vi "Slant.vi"(11 "GIC Input":T1={"     Use ?\nOff       On"=[FALSE, TRUE, FALSE, TRUE], "Mode:"=FALSE, "Extra Port"="", "Hokuyo Port"="COM7", "Tx Prop  Port"="COM6", "Compass Port"="", "GPS Port"="", "Num of WPs"=0, "WP Lats and Longs"={"WP Lats"=[], "WP Longs"=[]}, "Obst Lats and Longs"={"Obst Lats"=[], "Obst Longs"=[]}, "Parameters"=[], "GPS Data"=[], "Compass"=0.0, "LMS Vector"=[], "Vision Vector"=[], "Direction Cmd"=0.0, "Speed Cmd"=0.0, "WP Vector"=[], "WP Number"=0, "Extra"=0, "SW Map"=[], "Path Cluster"={"Path x node"=[], "Path y node"=[]}, "Sim Course"=[]} {"Obst Lats and Longs"."Obst Longs" format="%#_8g"; "Obst Lats and Longs"."Obst Lats" format="%#_8g"}) -> (3 "GIC Output":T1={"     Use ?\nOff       On"=[FALSE, TRUE, FALSE, TRUE], "Mode:"=FALSE, "Extra Port"="", "Hokuyo Port"="COM7", "Tx Prop  Port"="COM6", "Compass Port"="", "GPS Port"="", "Num of WPs"=0, "WP Lats and Longs"={"WP Lats"=[], "WP Longs"=[]}, "Obst Lats and Longs"={"Obst Lats"=[], "Obst Longs"=[]}, "Parameters"=[], "GPS Data"=[], "Compass"=0.0, "LMS Vector"=[], "Vision Vector"=[], "Direction Cmd"=0.0, "Speed Cmd"=0.0, "WP Vector"=[], "WP Number"=0, "Extra"=0, "SW Map"=[], "Path Cluster"={"Path x node"=[], "Path y node"=[]}, "Sim Course"=[]} {"Obst Lats and Longs"."Obst Longs" format="%#_8g"; "Obst Lats and Longs"."Obst Lats" format="%#_8g"})   [LabVIEW 2014]
panel:
  out "test1":dbl
  out "yy":dbl
  out "ll":dbl
  out "mm":dbl
  out "nn":dbl
  out "maxind":dbl
  out "maxi":dbl
  out "Test confidence":dbl
  out "Test slant":dbl
  in  "Test SWMap":i32[][](array[numeric])=array86x86[7396 elements]
  # "SLANT"
  # "Input:"
  # "Output"
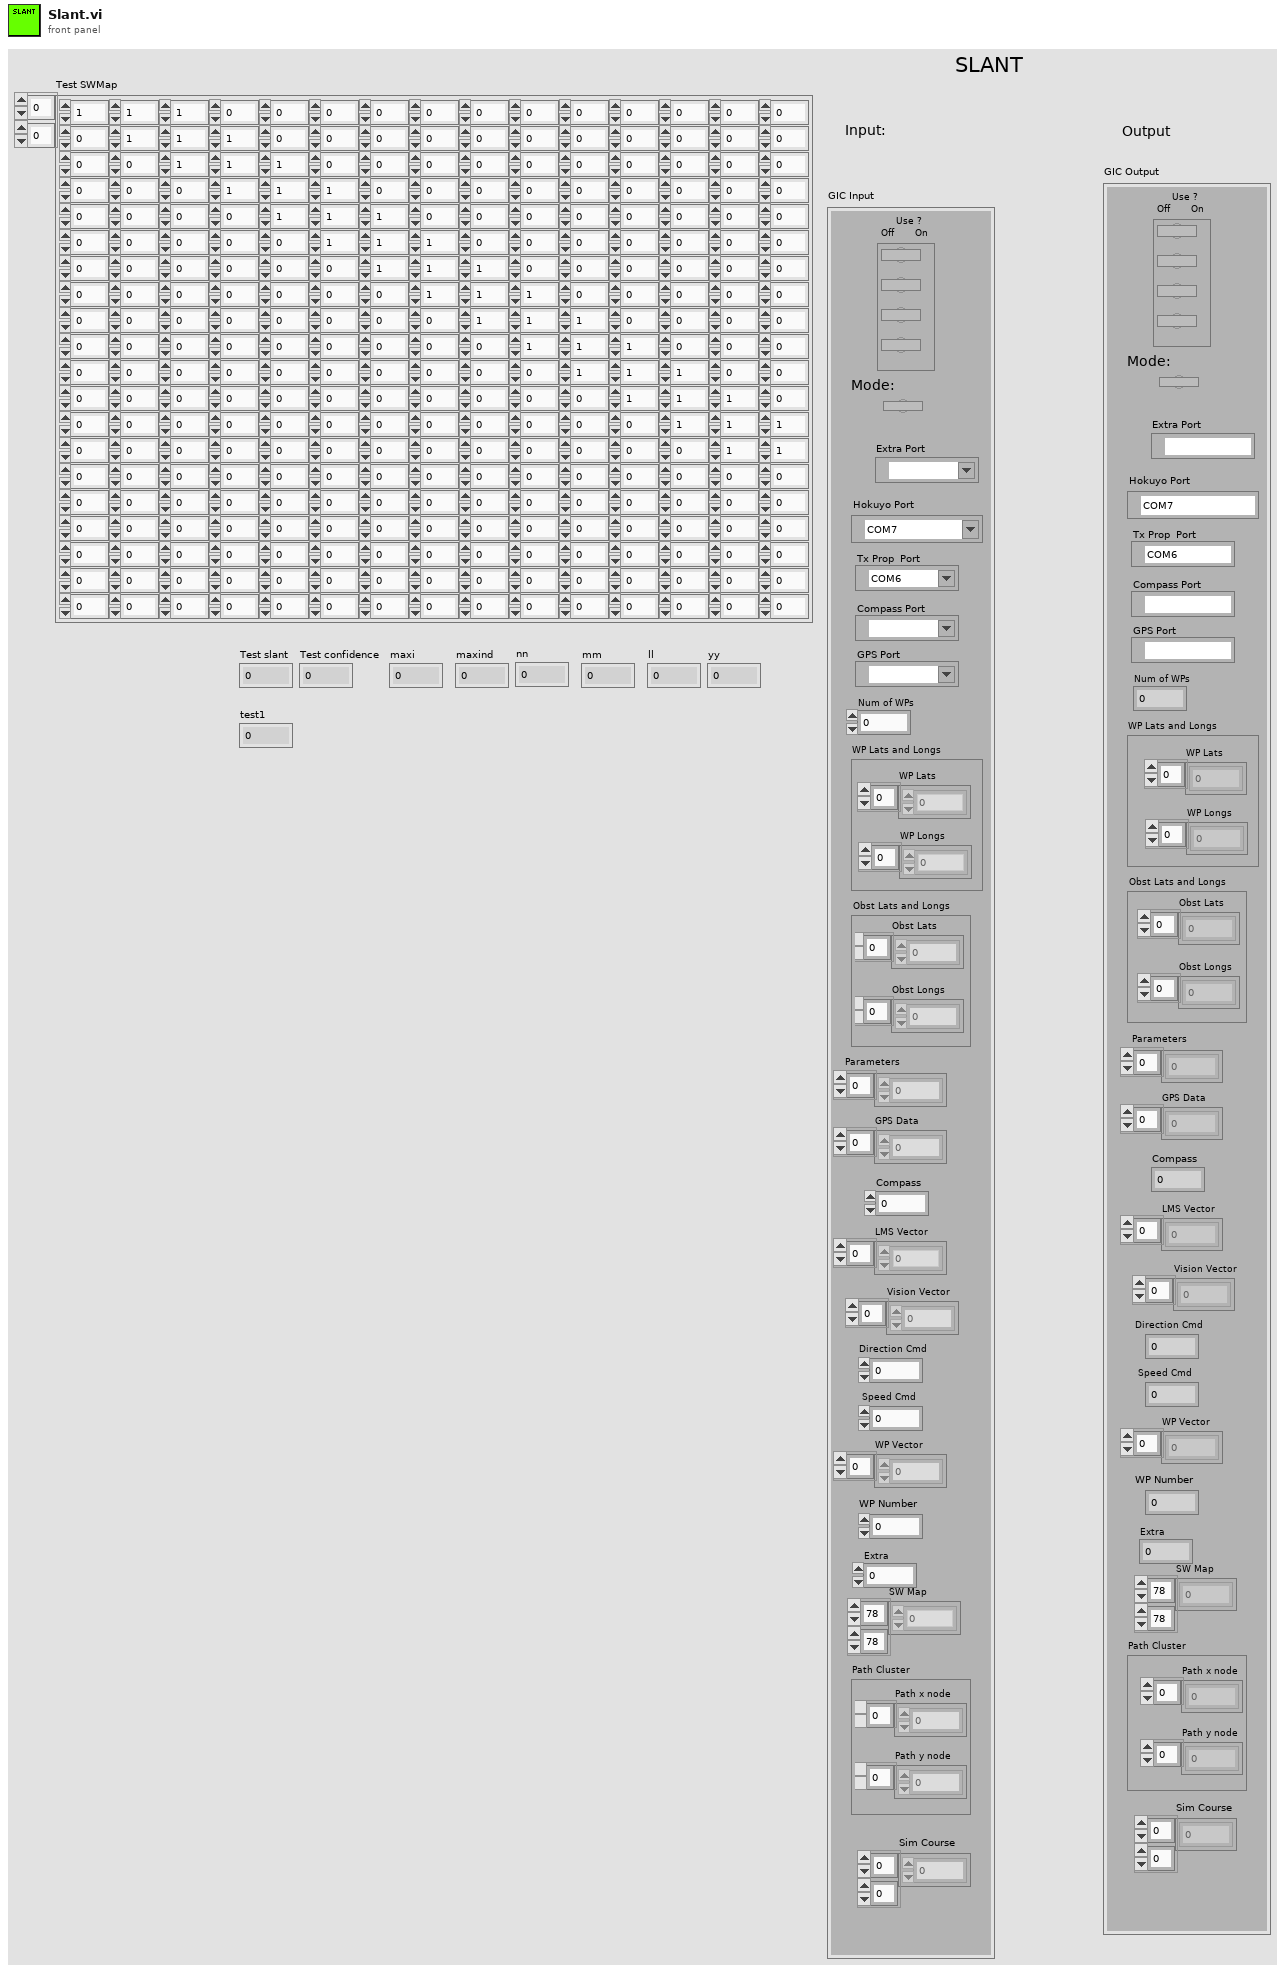
[diagram p1: front panel]
types:
  T1 = cluster{"     Use ?\nOff       On":bool[], "Mode:":bool, "Extra Port":refnum<visa-resource-name>, "Hokuyo Port":refnum<visa-resource-name>, "Tx Prop  Port":refnum<visa-resource-name>, "Compass Port":refnum<visa-resource-name>, "GPS Port":refnum<visa-resource-name>, "Num of WPs":i16, "WP Lats and Longs":cluster{"WP Lats":dbl[], "WP Longs":dbl[]}, "Obst Lats and Longs":cluster{"Obst Lats":dbl[], "Obst Longs":dbl[]}, "Parameters":dbl[], "GPS Data":dbl[], "Compass":dbl, "LMS Vector":dbl[], "Vision Vector":dbl[], "Direction Cmd":dbl, "Speed Cmd":dbl, "WP Vector":dbl[], "WP Number":i32, "Extra":i16, "SW Map":i32[][], "Path Cluster":cluster{"Path x node":dbl[], "Path y node":dbl[]}, "Sim Course":i8[][]}
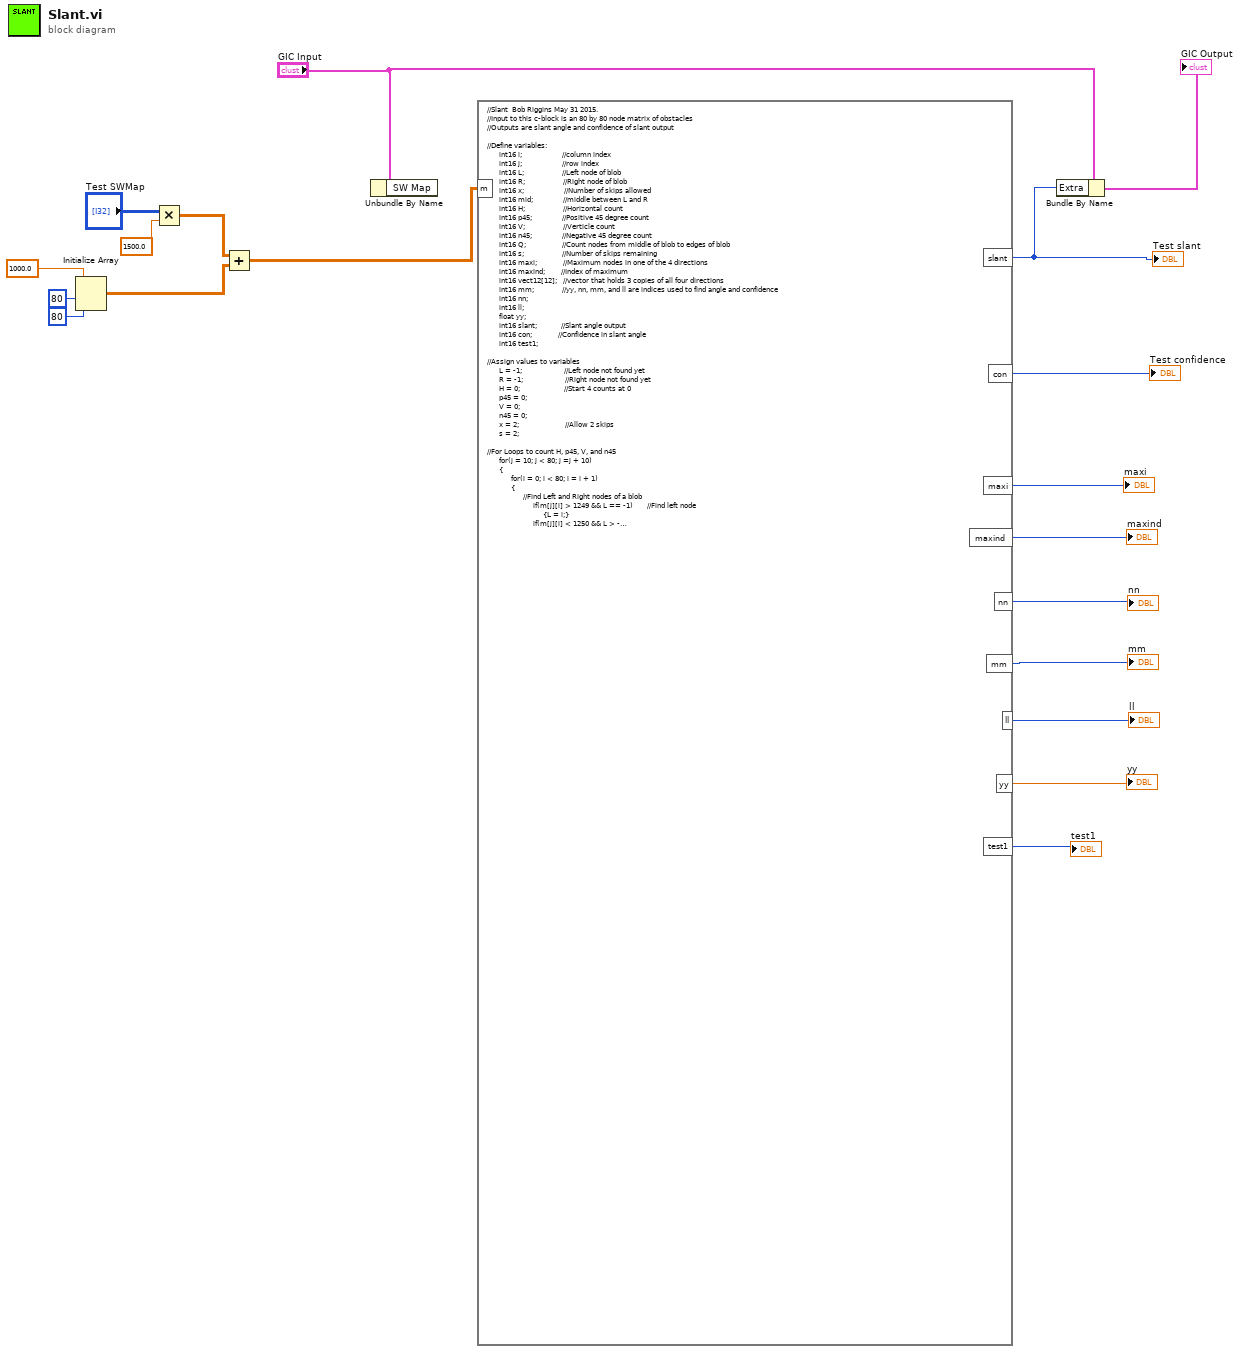
[diagram p0: block diagram]
diagram:
  n1 = Initialize Array(1000.0 ("element"), 80 ("dimension size"), 80 ("dimension size")) -> (w11:dbl[][])
  n2 = Multiply(x="Test SWMap", y=1500.0) -> (x*y=w12:dbl[][])
  n3 = Add(x=w12, y=w11) -> (x+y=w10:dbl[][])
  n4 = Unbundle By Name("GIC Input") -> ()  [unwired: 1 out]
  n5 = formula code="//Slant  Bob Riggins May 31 2015.  \n//Input to this c-block is an 80 by 80 node matrix of obstacles\n//Outputs are slant angle and confidence of slant output\n\n//Define variables:\n      int16 i;                    //column index\n      int16 j;                    //row index\n      int16 L;                   //Left node of blob\n      int16 R;                   //Right node of blob\n      int16 x;                    //Number of skips allowed\n      int16 mid;               //middle between L and R\n      int16 H;                   //Horizontal count\n      int16 p45;               //Positive 45 degree count\n      int16 V;                   //Verticle count\n      int16 n45;               //Negative 45 degree count\n      int16 Q;                  //Count nodes from middle of blob to edges of blob\n      int16 s;                   //Number of skips remaining\n      int16 maxi;             //Maximum nodes in one of the 4 directions\n      int16 maxind;        //Index of maximum\n      int16 vect12[12];   //vector that holds 3 copies of all four directions\n      int16 mm;              //yy, nn, mm, and ll are indices used to find angle and confidence\n      int16 nn;\n      int16 ll;\n      float yy;\n      int16 slant;            //Slant angle output\n      int16 con;             //Confidence in slant angle\n      int16 test1;\n\n//Assign values to variables\n      L = -1;                     //Left node not found yet\n      R = -1;                     //Right node not found yet\n      H = 0;                      //Start 4 counts at 0\n      p45 = 0;\n      V = 0;\n      n45 = 0;\n      x = 2;                       //Allow 2 skips\n      s = 2;\n\n//For Loops to count H, p45, V, and n45\n      for(j = 10; j < 80; j =j + 10)\n      {\n            for(i = 0; i < 80; i = i + 1)\n            {\n                  //Find Left and Right nodes of a blob\n                       if(m[j][i] > 1249 && L == -1)       //Find left node\n                            {L = i;}\n                       if(m[j][i] < 1250 && L > -1 && s == 0)          //Find right node\n                            {R = i - 1 - x;} \n                       if(m[j][i] <1250 && L > -1 && s > 0)         //Allow for skips\n                            {s = s - 1;}\n                       if(i == 79 && m[j][i] > 1249 && L == -1)      //single node at edge\n                       {                                                                            //define L and R there\n                             L == 79;\n                             R == 79;\n                       }       \n                       if(i == 79 && m[j][i] > 1249 && L > -1)       //blob at edge (L found)\n                            {R = 79;}   \n                       if(i == 79 && m[j][i] < 1250 && L > -1)       //blob at edge (L found)\n                            {R = 78;}\n\n                       if(L > -1 && R > -1)         //If L and R exist then start counting from mid\n                       {\n                            H = H + (R - L);                         //Updated H\n                            if(j==10)\n                                 {test1 = R;}\n                            mid = int((L + R)/2);                //Set up middle of blob for counting\n                            L = -1;\n                            R = -1;\n                            s = x;\n                            Q = 1; \n                \n                       //Count N45 (negative 45 degrees thru mid of blob)\n                            while (s > 0 && j + Q < 80 && mid + Q < 80)\n                                {\n                                     while (m[j + Q][mid + Q] > 1249)    //Count down and to right\n                                          {\n                                               n45 = n45 + 1;\n                                               s = x;\n                                               Q = Q + 1;\n                                          }\n                                     while (m[j + Q][mid + Q] < 1250 && s > 0)   //Allow x skips\n                                          {\n                                               n45 = n45 + 1;\n                                               s = s - 1;\n                                               Q = Q + 1;\n                                          }\n                                }     //end of while loop for counting n45 down and to right\n                                n45 = n45 - x;\n                                s = x;\n                                Q = 1;\n\n                                while (s > 0 && j - Q > -1 && mid - Q > -1)\n                                {\n                                     while (m[j - Q][mid - Q] > 1249)    //Count up and to left\n                                          {\n                                               n45 = n45 + 1;\n                                               s = x;\n                                               Q = Q + 1;\n                                          }\n                                     while (m[j - Q][mid - Q] < 1250 && s > 0)   //Allow x skips\n                                          {\n                                               n45 = n45 + 1;\n                                               s = s - 1;\n                                               Q = Q + 1;\n                                          }\n                                }     //end of while loop for counting n45 up and to left\n                                n45 = n45 - x;\n                                s = x;\n                                Q = 1;\n\n                       //Count V (verticle thru mid of blob)\n                            while (s > 0 && j + Q < 80)\n                                {\n                                     while (m[j + Q][mid] > 1249)    //Count down from mid\n                                          {\n                                               V = V + 1;\n                                               s = x;\n                                               Q = Q + 1;\n                                          }\n                                     while (m[j + Q][mid] < 1250 && s > 0)   //Allow x skips\n                                          {\n                                               V = V + 1;\n                                               s = s - 1;\n                                               Q = Q + 1;\n                                          }\n                                }     //end of while loop for counting V down\n                                V = V - x;\n                                s = x;\n                                Q = 1;\n\n                                while (s > 0 && j - Q > -1)\n                                {\n                                     while (m[j - Q][mid] > 1249)    //Count up\n                                          {\n                                               V = V + 1;\n                                               s = x;\n                                               Q = Q + 1;\n                                          }\n                                     while (m[j - Q][mid] < 1250 && s > 0)   //Allow x skips\n                                          {\n                                               V = V + 1;\n                                               s = s - 1;\n                                               Q = Q + 1;\n                                          }\n                                }     //end of while loop for counting V up\n                                V = V - x;\n                                s = x;\n                                Q = 1;\n\n                       //Count p45 (positive 45 degrees thru mid of blob)\n                            while (s > 0 && j + Q < 80 && mid - Q > -1)\n                                {\n                                     while (m[j + Q][mid - Q] > 1249)    //Count down and to left\n                                          {\n                                               p45 = p45 + 1;\n                                               s = x;\n                                               Q = Q + 1;\n                                          }\n                                     while (m[j + Q][mid - Q] < 1250 && s > 0)   //Allow x skips\n                                          {\n                                               p45 = p45 + 1;\n                                               s = s - 1;\n                                               Q = Q + 1;\n                                          }\n                                }     //end of while loop for counting p45 down and to left\n                                p45 = p45 - x;\n                                s = x;\n                                Q = 1;\n\n                                while (s > 0 && j - Q > -1 && mid + Q < 80)\n                                {\n                                     while (m[j - Q][mid + Q] > 1249)    //Count up and to right\n                                          {\n                                               p45 = p45 + 1;\n                                               s = x;\n                                               Q = Q + 1;\n                                          }\n                                     while (m[j - Q][mid + Q] < 1250 && s > 0)   //Allow x skips\n                                          {\n                                               p45 = p45 + 1;\n                                               s = s - 1;\n                                               Q = Q + 1;\n                                          }\n                                }     //end of while loop for counting p45 up and to right\n                                p45 = p45 - x;\n                                s = x;\n                                Q = 1;\n\n                       }                                                    //end of IF for counts for blob\n            }                                    //end of FOR for i\n      }                                          //end of FOR for j\n      \n      //Now have H, p45, V, n45.  Find slan and con  (slant angle and confidence)\n            maxi = H;                                   //Initialize process of finding maximum direction\n            maxind = 0;\n            if(p45 > maxi)\n            {\n                 maxi = p45;\n                 maxind = 1;\n            }\n            if(V > maxi)\n            {\n                 maxi = V;\n                 maxind = 2;\n            }\n            if(n45 > maxi)\n            {\n                 maxi = n45;\n                 maxind = 3;\n            }                                                    //now, max value of 4 directions in maxi\n                                                                 //maxind is index of direction of max\n\n            for(i = 0; i < 3; i = i + 1)            //Next, make vect12, 3 copies of 4 directions\n            {\n                 vect12[4*i] = H;\n                 vect12[4*i + 1] = p45;\n                 vect12[4*i + 2] = V;\n                 vect12[4*i + 3] = n45;\n            }\n           \n            if(maxi != 0)\n            {\n                 nn = vect12[maxind - 1];                          //Use max direction and \"pull\" off to sides\n                 mm = vect12[maxind + 1];\n                 ll = vect12[maxind + 2];\n                 yy = (mm - nn)/(maxi + mm + mm);\n                 con = (1 - (ll/maxi)) * 100;                                    //Confidence of slant calculation\n\n                 if(maxind == 0)                                         //Find slant angle\n                    {slant = 45 * yy;}\n                 if(maxind == 1)                                         \n                    {slant = 45 * (1 - yy);}\n                 if(maxind == 2)                                         \n                    {slant = (45 * (1 - yy)) - 45;}\n                 if(maxind == 3)                                         \n                    {slant = -45 * (1 + yy);}\n             }\n\n             if(maxi == 0)\n             {\n                  slant = 0;\n                  con = 0;\n             }"("m"=w10) -> ("slant"=w9:i16, "con"=→"Test confidence":i16, "maxi"=→"maxi":i16, "maxind"=→"maxind":i16, "nn"=→"nn":i16, "mm"=→"mm":i16, "ll"=→"ll":i16, "yy"=→"yy":dbl, "test1"=→"test1":i16)
  "Test slant" <- w9
  n6 = Bundle By Name(cluster="GIC Input", "Extra"=w9) -> (→"GIC Output":T1)
